vi "Data_Validation.vi"(11 "Array":dbl[][](array[numeric])) -> (3 "Correct Record":bool)   [LabVIEW 2020]
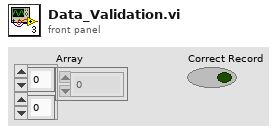
[diagram p1: front panel]
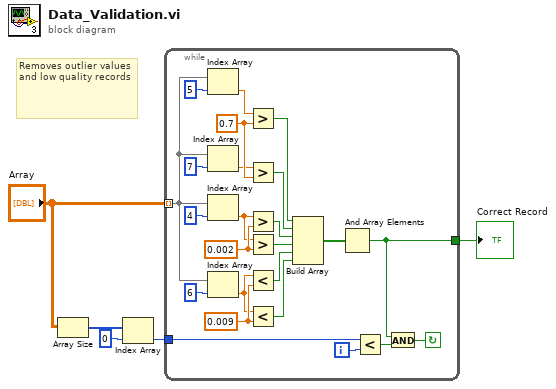
[diagram p0: block diagram]
diagram:
  # "Removes outlier values and low quality records"
  n1 = Array Size(array="Array") -> (size(s)=w1:i32[])
  n2 = Index Array(array=w1, index=0) -> (element=w3:i32)
  n3 = while {
    tunnel: "Array" -> [w6] mode=indexing
    tunnel: w3 -> [w14]
    tunnel: [w8] -> w5
    i -> [w7]
    stop <- w12 continue-if-true
    w10 = 0.002
    w22 = 0.009
    w26 = 0.7
    n4 = Index Array(array=w6, index=5) -> (element=w28:dbl)
    n5 = Index Array(array=w6, index=7) -> (element=w25:dbl)
    n6 = Index Array(array=w6, index=4) -> (element=w9:dbl)
    n7 = Index Array(array=w6, index=6) -> (element=w11:dbl)
    n8 = Greater?(x=w28, y=w26) -> (0:w21:bool)
    n9 = Greater?(x=w25, y=w26) -> (0:w20:bool)
    n10 = Greater?(x=w9, y=w10) -> (0:w19:bool)
    n11 = Greater?(x=w9, y=w10) -> (0:w18:bool)
    n12 = Less?(x=w11, y=w22) -> (x < y?=w17:bool)
    n13 = Less?(x=w11, y=w22) -> (x < y?=w16:bool)
    n14 = Build Array(w21, w20, w19, w18, w17, w16) -> (w15:bool[])
    n15 = And Array Elements(Boolean array=w15) -> (logical AND=w8:bool)
    n16 = Less?(x=w14, y=w7) -> (x < y?=w13:bool)
    n17 = And(x=w8, y=w13) -> (x .and. y?=w12:bool)
  }
  "Correct Record" <- w5
